vi "Kalman G.vi"(10 "intervalo":dbl=1.0) -> (2 "G":dbl[][](array[numeric]))   [LabVIEW 2023]
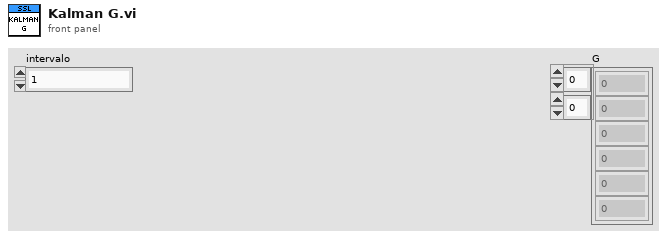
[diagram p1: front panel]
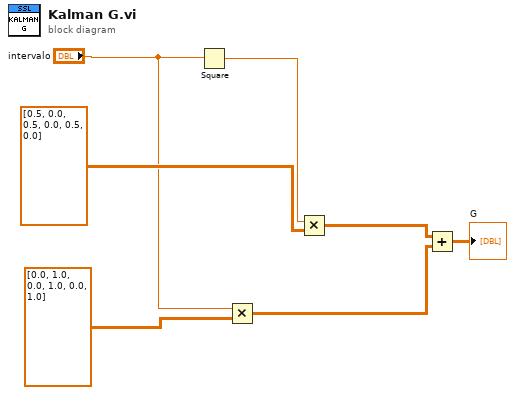
[diagram p0: block diagram]
diagram:
  n1 = Square(x="intervalo") -> (x^2=w7:dbl)
  n2 = Multiply(x="intervalo", y=dbl[][] [[0.0], [1.0], [0.0], [1.0], [0.0], [1.0]]) -> (x*y=w2:dbl[][])
  n3 = Multiply(x=w7, y=dbl[][] [[0.5], [0.0], [0.5], [0.0], [0.5], [0.0]]) -> (x*y=w5:dbl[][])
  n4 = Add(x=w5, y=w2) -> (x+y=→"G":dbl[][])
